vi "Bytes at port comparsion.vi"(8 "error in (no error)":errorcluster, 9 "x":u32=10, 11 "VISA Refnum in":refnum<visa-resource-name>) -> (0 "error out":errorcluster, 1 "bytes more then X ?":bool, 2 "Bytes at Port":u32, 3 "VISA Refnum out":refnum<visa-resource-name>)   [LabVIEW 2012]
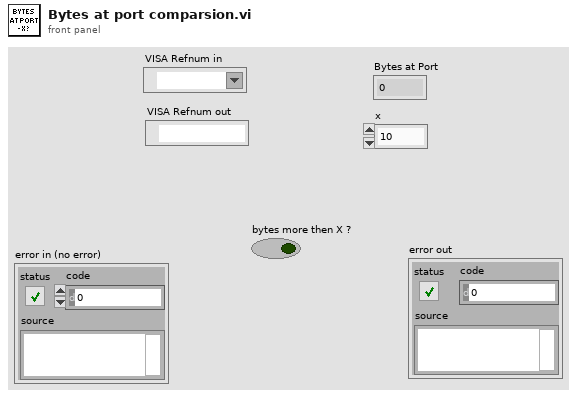
[diagram p1: front panel]
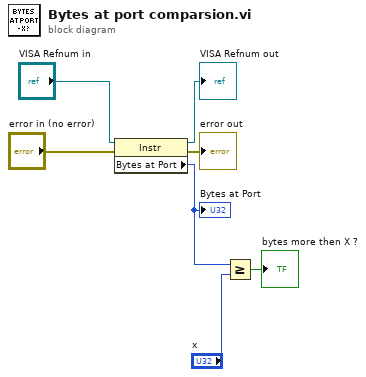
[diagram p0: block diagram]
diagram:
  n1 = property class="Instr"(reference="VISA Refnum in", error in="error in (no error)") -> (reference out=→"VISA Refnum out":refnum<visa-resource-name>, error out=→"error out":errorcluster, "Bytes at Port"=w7:u32)
  "Bytes at Port" <- w7
  n2 = Greater Or Equal?(x=w7, y="x") -> (x >= y?=→"bytes more then X ?":bool)
